vi "Plate Configuration_new_new.vi"(7 "all rows":string[][](array[string])=[["", "Well", "Fluor", "Target", "Content", "Sample", "Cq", "SQ"], ["", "A01", "SYBR", "Fos", "Unkn", "Fl1", "23.40", ""], ["", "A02", "SYBR", "Fos", "Unkn", "Fl1", "23.24", ""], ["", "A03", "SYBR", "Fos", "Unkn", "Fl2", "23.55", ""], ["", "A04", "SYBR", "Fos", "Unkn", "Fl2", "23.53", ""], ["", "A05", "SYBR", "Fos", "Unkn", "Fl3", "23.38", ""], ["", "A06", "SYBR", "Fos", "Unkn", "Fl3", "23.50", ""], ["", "A07", "SYBR", "Fos", "Unkn", "Pfl1", "22.43", ""], ["", "A08", "SYBR", "Fos", "Unkn", "Pfl1", "22.94", ""], ["", "A09", "SYBR", "Fos", "Unkn", "Pfl2", "21.10", ""], ["", "A10", "SYBR", "Fos", "Unkn", "Pfl2", "21.46", ""], ["", "A11", "SYBR", "Fos", "Unkn", "Pfl3", "22.49", ""], ["", "A12", "SYBR", "Fos", "Unkn", "Pfl3", "22.89", ""], ["", "B01", "SYBR", "Arc", "Unkn", "Fl1", "32.28", ""], ["", "B02", "SYBR", "Arc", "Unkn", "Fl1", "32.59", ""], ["", "B03", "SYBR", "Arc", "Unkn", "Fl2", "32.93", ""], ["", "B04", "SYBR", "Arc", "Unkn", "Fl2", "32.78", ""], ["", "B05", "SYBR", "Arc", "Unkn", "Fl3", "32.38", ""], ["", "B06", "SYBR", "Arc", "Unkn", "Fl3", "32.35", ""], ["", "B07", "SYBR", "Arc", "Unkn", "Pfl1", "30.44", ""], ["", "B08", "SYBR", "Arc", "Unkn", "Pfl1", "30.58", ""], ["", "B09", "SYBR", "Arc", "Unkn", "Pfl2", "30.07", ""], ["", "B10", "SYBR", "Arc", "Unkn", "Pfl2", "30.20", ""], ["", "B11", "SYBR", "Arc", "Unkn", "Pfl3", "30.38", ""], ["", "B12", "SYBR", "Arc", "Unkn", "Pfl3", "30.04", ""], ["", "C01", "SYBR", "Jun", "Unkn", "Fl1", "25.27", ""], ["", "C02", "SYBR", "Jun", "Unkn", "Fl1", "24.72", ""], ["", "C03", "SYBR", "Jun", "Unkn", "Fl2", "25.47", ""], ["", "C04", "SYBR", "Jun", "Unkn", "Fl2", "25.79", ""], ["", "C05", "SYBR", "Jun", "Unkn", "Fl3", "25.27", ""], ["", "C06", "SYBR", "Jun", "Unkn", "Fl3", "25.52", ""], ["", "C07", "SYBR", "Jun", "Unkn", "Pfl1", "23.53", ""], ["", "C08", "SYBR", "Jun", "Unkn", "Pfl1", "23.37", ""], ["", "C09", "SYBR", "Jun", "Unkn", "Pfl2", "21.29", ""], ["", "C10", "SYBR", "Jun", "Unkn", "Pfl2", "38.35", ""], ["", "C11", "SYBR", "Jun", "Unkn", "Pfl3", "23.20", ""], ["", "C12", "SYBR", "Jun", "Unkn", "Pfl3", "23.23", ""], ["", "D01", "SYBR", "JunB", "Unkn", "Fl1", "26.08", ""], ["", "D02", "SYBR", "JunB", "Unkn", "Fl1", "26.09", ""], ["", "D03", "SYBR", "JunB", "Unkn", "Fl2", "27.02", ""], ["", "D04", "SYBR", "JunB", "Unkn", "Fl2", "27.08", ""], ["", "D05", "SYBR", "JunB", "Unkn", "Fl3", "26.91", ""], ["", "D06", "SYBR", "JunB", "Unkn", "Fl3", "26.93", ""], ["", "D07", "SYBR", "JunB", "Unkn", "Pfl1", "25.32", ""], ["", "D08", "SYBR", "JunB", "Unkn", "Pfl1", "25.12", ""], ["", "D09", "SYBR", "JunB", "Unkn", "Pfl2", "24.28", ""], ["", "D10", "SYBR", "JunB", "Unkn", "Pfl2", "24.21", ""], ["", "D11", "SYBR", "JunB", "Unkn", "Pfl3", "25.01", ""], ["", "D12", "SYBR", "JunB", "Unkn", "Pfl3", "25.38", ""], ["", "E01", "SYBR", "Ctgf", "Unkn", "Fl1", "27.57", ""], ["", "E02", "SYBR", "Ctgf", "Unkn", "Fl1", "27.52", ""], ["", "E03", "SYBR", "Ctgf", "Unkn", "Fl2", "28.24", ""], ["", "E04", "SYBR", "Ctgf", "Unkn", "Fl2", "28.02", ""], ["", "E05", "SYBR", "Ctgf", "Unkn", "Fl3", "28.10", ""], ["", "E06", "SYBR", "Ctgf", "Unkn", "Fl3", "27.90", ""], ["", "E07", "SYBR", "Ctgf", "Unkn", "Pfl1", "25.17", ""], ["", "E08", "SYBR", "Ctgf", "Unkn", "Pfl1", "25.51", ""], ["", "E09", "SYBR", "Ctgf", "Unkn", "Pfl2", "25.49", ""], ["", "E10", "SYBR", "Ctgf", "Unkn", "Pfl2", "25.43", ""], ["", "E11", "SYBR", "Ctgf", "Unkn", "Pfl3", "25.45", ""], ["", "E12", "SYBR", "Ctgf", "Unkn", "Pfl3", "25.45", ""], ["", "F01", "SYBR", "Nr4a1", "Unkn", "Fl1", "25.09", ""], ["", "F02", "SYBR", "Nr4a1", "Unkn", "Fl1", "25.24", ""], ["", "F03", "SYBR", "Nr4a1", "Unkn", "Fl2", "26.15", ""], ["", "F04", "SYBR", "Nr4a1", "Unkn", "Fl2", "26.01", ""], ["", "F05", "SYBR", "Nr4a1", "Unkn", "Fl3", "26.17", ""], ["", "F06", "SYBR", "Nr4a1", "Unkn", "Fl3", "26.29", ""], ["", "F07", "SYBR", "Nr4a1", "Unkn", "Pfl1", "24.23", ""], ["", "F08", "SYBR", "Nr4a1", "Unkn", "Pfl1", "24.26", ""], ["", "F09", "SYBR", "Nr4a1", "Unkn", "Pfl2", "23.05", ""], ["", "F10", "SYBR", "Nr4a1", "Unkn", "Pfl2", "23.08", ""], ["", "F11", "SYBR", "Nr4a1", "Unkn", "Pfl3", "24.02", ""], ["", "F12", "SYBR", "Nr4a1", "Unkn", "Pfl3", "24.04", ""], ["", "G01", "SYBR", "Egr1", "Unkn", "Fl1", "26.85", ""], ["", "G02", "SYBR", "Egr1", "Unkn", "Fl1", "26.59", ""], ["", "G03", "SYBR", "Egr1", "Unkn", "Fl2", "27.75", ""], ["", "G04", "SYBR", "Egr1", "Unkn", "Fl2", "27.76", ""], ["", "G05", "SYBR", "Egr1", "Unkn", "Fl3", "27.92", ""], ["", "G06", "SYBR", "Egr1", "Unkn", "Fl3", "28.27", ""], ["", "G07", "SYBR", "Egr1", "Unkn", "Pfl1", "25.19", ""], ["", "G08", "SYBR", "Egr1", "Unkn", "Pfl1", "24.90", ""], ["", "G09", "SYBR", "Egr1", "Unkn", "Pfl2", "23.36", ""], ["", "G10", "SYBR", "Egr1", "Unkn", "Pfl2", "23.81", ""], ["", "G11", "SYBR", "Egr1", "Unkn", "Pfl3", "24.67", ""], ["", "G12", "SYBR", "Egr1", "Unkn", "Pfl3", "24.81", ""], ["", "H01", "SYBR", "beta-Actin", "Unkn", "Fl1", "22.22", ""], ["", "H02", "SYBR", "beta-Actin", "Unkn", "Fl1", "22.27", ""], ["", "H03", "SYBR", "beta-Actin", "Unkn", "Fl2", "22.94", ""], ["", "H04", "SYBR", "beta-Actin", "Unkn", "Fl2", "22.82", ""], ["", "H05", "SYBR", "beta-Actin", "Unkn", "Fl3", "23.04", ""], ["", "H06", "SYBR", "beta-Actin", "Unkn", "Fl3", "22.72", ""], ["", "H07", "SYBR", "beta-Actin", "Unkn", "Pfl1", "22.09", ""], ["", "H08", "SYBR", "beta-Actin", "Unkn", "Pfl1", "22.09", ""], ["", "H09", "SYBR", "beta-Actin", "Unkn", "Pfl2", "21.57", ""], ["", "H10", "SYBR", "beta-Actin", "Unkn", "Pfl2", "21.16", ""], ["", "H11", "SYBR", "beta-Actin", "Unkn", "Pfl3", "21.80", ""], ["", "H12", "SYBR", "beta-Actin", "Unkn", "Pfl3", "21.93", ""]] caption="모든 행") -> (0 "출력 클러스터":T4, 1 "RowHdrs":string[](array[string]), 2 "Internal Ctrl":string[][](array[string]), 3 "Target Gene":string[][][](array[string]))   [LabVIEW 2017]
panel:
  in  "12":string="KO3"
  in  "11":string="KO3"
  in  "10":string="WT3"
  in  "09":string="WT3"
  in  "08":string="KO2"
  in  "07":string="KO2"
  in  "06":string="WT2"
  in  "05":string="WT2"
  in  "04":string="KO1"
  in  "03":string="KO1"
  in  "02":string="WT1"
  in  "01":string="WT1"
  in  "ColLabel":T1(array[ring])=[enum."11", enum."11", enum."21", enum."21", enum."12", enum."12", enum."22", enum."22", enum."13", enum."13", enum."23", enum."23"]
  out "RowLabel":T2(array[cluster])
  in  "H":string="H"
  in  "G":string="G"
  in  "F":string="F"
  in  "E":string="E"
  in  "D":string="D"
  in  "C":string="C"
  in  "B":string="B"
  in  "RowLabel":T3(array[ring])
  in  "A":string="A"
  in  "출력 클러스터 2":T4={"Group #"=2.0, "Biological replicate"=3.0, "Technical replicate"=2.0}
  out "ColLabel (C)":T5(array[cluster])=[{"ColNames"="01", "Label"=enum."11"}, {"ColNames"="02", "Label"=enum."11"}, {"ColNames"="03", "Label"=enum."12"}, {"ColNames"="04", "Label"=enum."12"}, {"ColNames"="05", "Label"=enum."13"}, {"ColNames"="06", "Label"=enum."13"}, {"ColNames"="07", "Label"=enum."21"}, {"ColNames"="08", "Label"=enum."21"}, {"ColNames"="09", "Label"=enum."22"}, {"ColNames"="10", "Label"=enum."22"}, {"ColNames"="11", "Label"=enum."23"}, {"ColNames"="12", "Label"=enum."23"}]
  in  "정지":bool
  # "Sample"
  # "Label"
  # "Gene Name"
  # "Label"
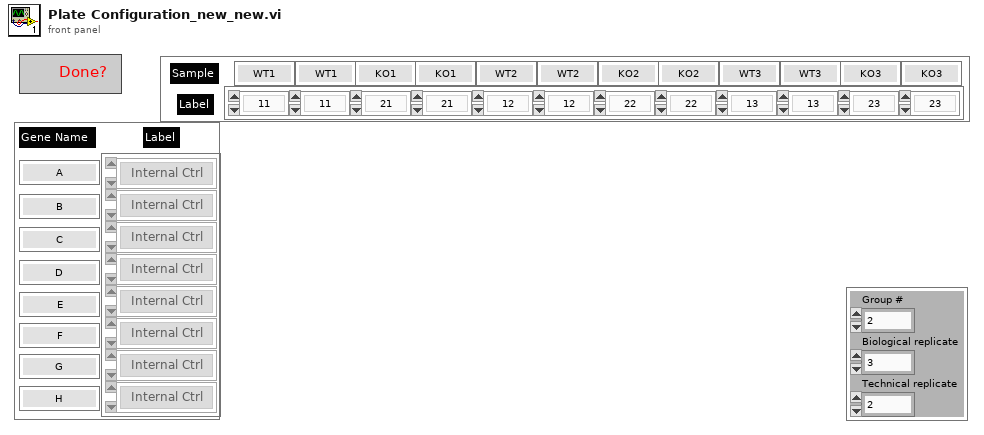
[diagram p1: front panel]
types:
  T1 = enum16{"11", "12", "13", "21", "22", "23", "Empty"}[]
  T2 = cluster{"H":string, "Label":enum16{"Empty Ch", "Target Ch", "Internal Ctrl"}}[]
  T3 = enum16{"Empty Ch", "Target Ch", "Internal Ctrl"}[]
  T4 = cluster{"Group #":dbl, "Biological replicate":dbl, "Technical replicate":dbl}
  T5 = cluster{"ColNames":string, "Label":enum16{"11", "12", "13", "21", "22", "23", "Empty"}}[]
  T6 = cluster{"H":string, "Label":enum16{"Empty Ch", "Target Ch", "Internal Ctrl"}}
  T7 = cluster{"12":string, "Label":enum16{"11", "12", "13", "21", "22", "23", "Empty"}}
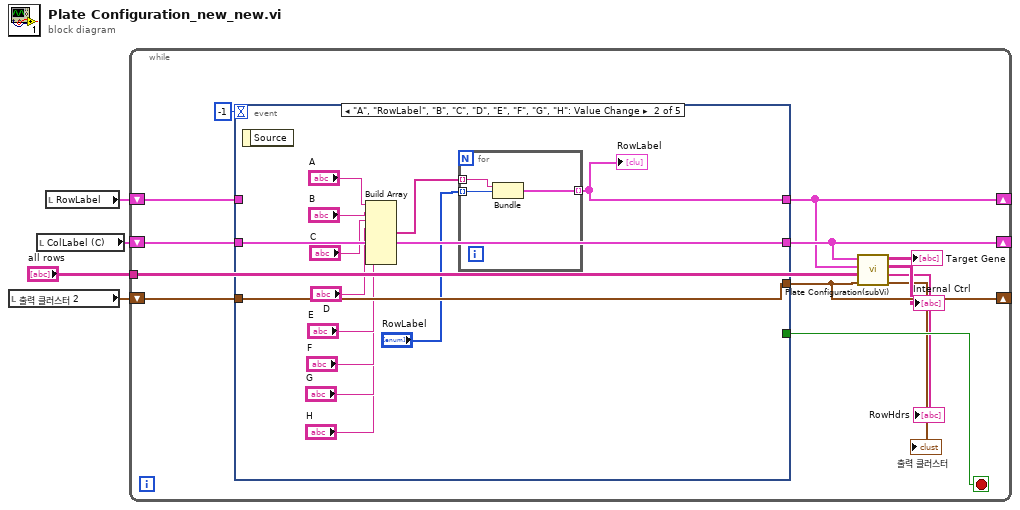
[diagram p0: block diagram]
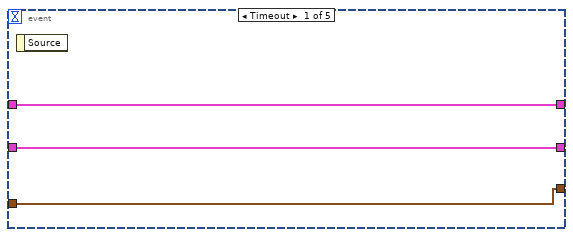
[diagram p2: hidden frame]
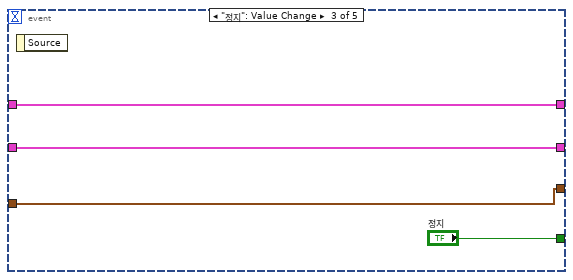
[diagram p3: hidden frame]
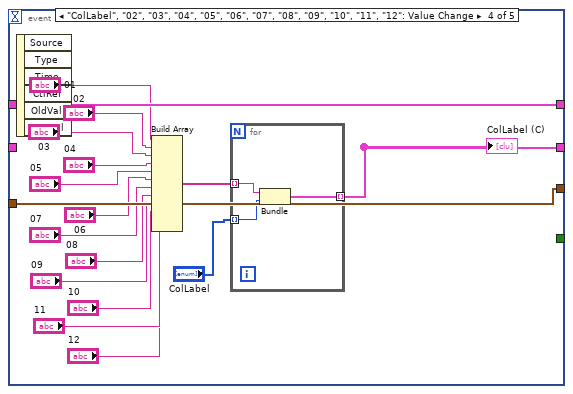
[diagram p4: hidden frame]
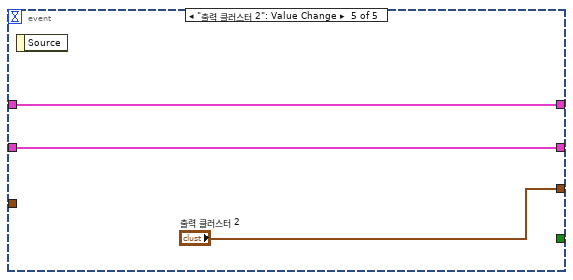
[diagram p5: hidden frame]
diagram:
  n1 = local read "출력 클러스터 2"() -> (w2:T4)
  n2 = local read "ColLabel (C)"() -> (w3:T5)
  n3 = local read "RowLabel"() -> (w1:T2)
  n4 = while {
    shift-right: [w12] -> _
    shift-left: w1 -> [w16]
    shift-right: [w13] -> _
    shift-left: w3 -> [w15]
    shift-right: [w11] -> _
    shift-left: w2 -> [w10]
    tunnel: "all rows" -> [w5]
    stop <- w14 stop-if-true
    n5 = event shown="[1] \"A\", \"RowLabel\", \"B\", \"C\", \"D\", \"E\", \"F\", \"G\", \"H\": Value Change" {
      selector: _ -> [_ _ _ _ _]
      dyn-events: _ -> [_ _ _ _ _]
      timeout: -1 -> [_ _ _ _ _]
      tunnel: [w20 w21 w39 w57 w63] -> w12
      tunnel: [w19 w33 w38 w41 w62] -> w13
      tunnel: w16 -> [w20 _ w39 w57 w63]
      tunnel: w15 -> [w19 w33 w38 _ w62]
      tunnel: [_ _ "정지" _ _] -> w14
      tunnel: [w18 w32 w37 w56 "출력 클러스터 2"] -> w11
      tunnel: w10 -> [w18 w32 w37 w56 _]
      event Timeout {
        n6 = event-data() -> ()  [unwired: 1 in, 1 out]
      }
      event "A", "RowLabel", "B", "C", "D", "E", "F", "G", "H": Value Change {
        n7 = event-data() -> ()  [unwired: 1 in, 1 out]
        n8 = Build Array("A", "B", "C", "D", "E", "F", "G", "H") -> (w23:string[])
        n9 = for {
          tunnel: w23 -> [w36] mode=indexing
          tunnel: "RowLabel" -> [w35] mode=indexing
          tunnel: [w34] -> w21 mode=indexing
          n10 = Bundle("H"=w36, "Label"=w35) -> (w34:T6)  [unwired: 1 in]
        }
        "RowLabel" <- w21
      }
      event "정지": Value Change {
        n11 = event-data() -> ()  [unwired: 1 in, 1 out]
      }
      event "ColLabel", "02", "03", "04", "05", "06", "07", "08", "09", "10", "11", "12": Value Change {
        n12 = event-data() -> ()  [unwired: 1 in, 6 out]
        n13 = Build Array("01", "02", "03", "04", "05", "06", "07", "08", "09", "10", "11", "12") -> (w42:string[])
        n14 = for {
          tunnel: "ColLabel" -> [w59] mode=indexing
          tunnel: w42 -> [w60] mode=indexing
          tunnel: [w58] -> w41 mode=indexing
          n15 = Bundle("12"=w60, "Label"=w59) -> (w58:T7)  [unwired: 1 in]
        }
        "ColLabel (C)" <- w41
      }
      event "출력 클러스터 2": Value Change {
        n16 = event-data() -> ()  [unwired: 1 in, 1 out]
      }
    }
    n17 = call "Plate Configuration(subVi).vi"("출력 클러스터 2"=w11, "all rows"=w5, "RowLabel"=w12, "ColLabel"=w13) -> ("출력 클러스터"=→"출력 클러스터":T4, "RowHdrs"=→"RowHdrs":string[], "Internal Ctrl"=→"Internal Ctrl":string[][], "Target Gene"=→"Target Gene":string[][][])
  }
